vi "ctx allocate new context.vi"() -> (3 "function return":u32)   [LabVIEW 2019, in "apdm.lvlib"]
doc: "APDM_EXPORT apdm_ctx_t apdm_ctx_allocate_new_context(void);"
uses:
  apdm.lvlib
  Lee Lab/CP FES Walking 2018/Code/Working/LabVIEW/apdm.dll
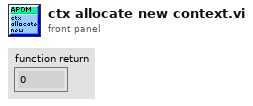
[diagram p1: front panel]
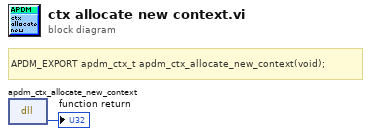
[diagram p0: block diagram]
diagram:
  # "APDM_EXPORT apdm_ctx_t apdm_ctx_allocate_new_context(void);"
  n1 = dll-call lib="C:/Users/jfalesi/Dropbox/Lee Lab/CP FES Walking 2018/Code/Working/LabVIEW/apdm.*" fn="apdm_ctx_allocate_new_context"() -> (→"function return":u32)  [unwired: 3 in, 2 out]
